vi "Measure.vi"(8 "error in (no error)":errorcluster, 9 "measurement configuration":variant, 10 "measure call context in":refnum<class "Measure Call Context.lvclass">, 11 "measurement plugin in":refnum<class "Automotive-Ethernet.lvclass">) -> (0 "error out":errorcluster, 1 "measurement results":variant, 2 "measure call context out":refnum<class "Measure Call Context.lvclass">, 3 "measurement plugin out":refnum<class "Automotive-Ethernet.lvclass">)   [LabVIEW 2025, in "Automotive-Ethernet.lvclass"]
uses:
  Automotive-Ethernet.lvclass
  <vilib>/Plug-In SDKs/Measurements/Measure Call Context/Measure Call Context.lvclass
  Measurement Configuration.ctl
  Automotive-Ethernet.lvclass/Automotive-Ethernet.ctl
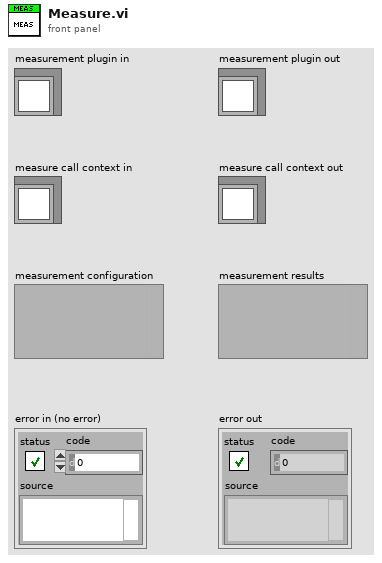
[diagram p1: front panel]
types:
  T1 = typedef "Automotive-Ethernet.lvclass/Measurement Configuration.ctl" = cluster{"double array in":dbl[], "double in":dbl, "U32 array in":u32[], "U32 in":u32, "U64 array in":u64[], "U64 in":u64, "I32 array in":i32[], "I32 in":i32, "I64 array in":i64[], "I64 in":i64, "bool in":bool, "string in":string, "u32 color ring in":u32, "u32 animal enum in":enum32{"Rabbit", "Gopher", "Badger"}}
  T2 = typedef "Automotive-Ethernet.lvclass/Measurement Results.ctl" = cluster{"xy data out":T3, "double array out":dbl[], "double out":dbl, "U32 array out":u32[], "U32 out":u32, "U64 array out":u64[], "U64 out":u64, "I32 array out":i32[], "I32 out":i32, "I64 array out":i64[], "I64 out":i64, "bool out":bool, "string out":string, "u32 color ring out":u32, "u32 animal enum out":enum32{"Rabbit", "Gopher", "Badger"}}
  T3 = typedef "ni.protobuf.types.lvlib/ni_protobuf_types_DoubleXYData.ctl" = cluster{"x_data":dbl[], "y_data":dbl[]}
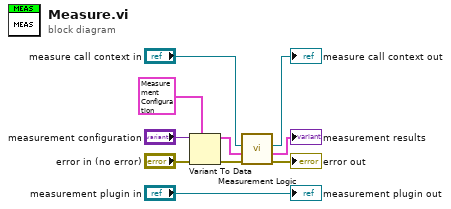
[diagram p0: block diagram]
diagram:
  n1 = Variant To Data(error in="error in (no error)", type=T1 {"double array in"=[3.4, 5.6], "double in"=1.2, "U32 array in"=[32, 33], "U32 in"=32, "U64 array in"=[64, 65], "U64 in"=64, "I32 array in"=[-32, -33], "I32 in"=-32, "I64 array in"=[-64, -65], "I64 in"=-64, "bool in"=TRUE, "string in"="Lorem ipsum dolor sit", "u32 color ring in"=1, "u32 animal enum in"=enum."Gopher"} ("measurement configuration"), Variant="measurement configuration") -> (data=w1:T1, error out=w7:errorcluster)
  n2 = call "Measurement Logic.vi"("error in"=w7, "measurement configuration"=w1, "measure call context in"="measure call context in") -> ("error out"=→"error out":errorcluster, "measurement results"=→"measurement results":T2, "measure call context out"=→"measure call context out":refnum<class "Measure Call Context.lvclass">)  [unwired: 6 in]
  "measurement plugin out" <- "measurement plugin in"
